vi "Write Attribute Types.vi"(10 "Attribute Types":string[](array[string]), 11 "Sequence Dialog in":refnum<class "Sequence Dialog.lvclass">) -> (3 "Sequence Dialog out":refnum<class "Sequence Dialog.lvclass">)   [LabVIEW 2017, in "Sequence Dialog.lvclass"]
uses:
  <vilib>/gpm_packages/@cs/Test-executive-builder/Source/Test Executive Builder Dialogs/Edit Sequence Dialog/Sequence Dialog.lvclass
  <vilib>/gpm_packages/@cs/Test-executive-builder/Source/Test Executive Builder Dialogs/Edit Sequence Dialog/Sequence Dialog.lvclass/Sequence Dialog.ctl
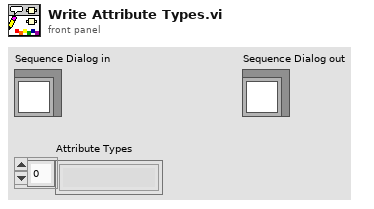
[diagram p1: front panel]
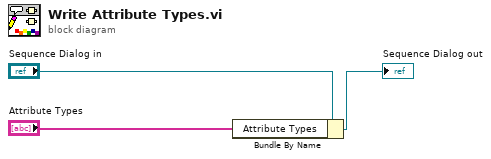
[diagram p0: block diagram]
diagram:
  n1 = Bundle By Name(cluster="Sequence Dialog in", "Attribute Types"="Attribute Types") -> (→"Sequence Dialog out":refnum<class "Sequence Dialog.lvclass">)
